vi "simple get func.vi"(11 "parameters":variant) -> (1 "error":errorcluster, 2 "data":variant, 3 "data ID":string)   [LabVIEW 2015]
uses:
  <vilib>/httpClient/LabVIEWHTTPClient.lvlib
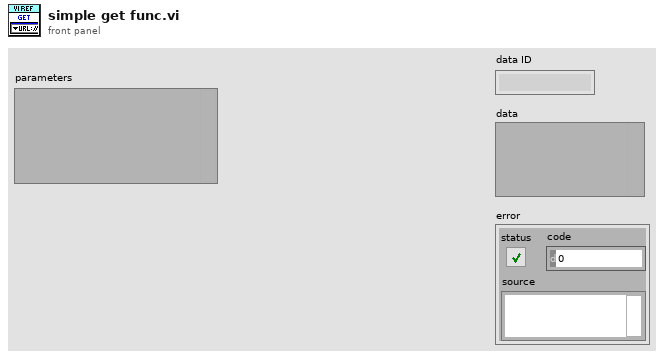
[diagram p1: front panel]
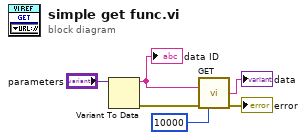
[diagram p0: block diagram]
diagram:
  n1 = Variant To Data(Variant="parameters") -> (data=w2:string, error out=w3:errorcluster)  [unwired: 2 in]
  "data ID" <- w2
  n2 = call <vilib>:"GET.vi"("url"=w2, "error in (no error)"=w3, "timeout (10000)"=10000) -> ("body"=→"data":string, "error out"=→"error":errorcluster)  [unwired: 9 in, 2 out]
